vi "stimulate3.vi"(4 "Injection point":T3, 6 "Stimulus":sgl[](array[numeric])=[0.0, 0.0, 0.0, 0.0, 0.0, 0.0] format="%#_3p", 7 "Input 1":sgl[](array[numeric])=[0.0, 0.0, 0.0] format="%#_3p", 8 "Input 0":sgl[](array[numeric])=[0.0, 0.0, 0.0] format="%#_3p", 10 "Parameters":T1={"Stimulus"={"Type"=enum."Off", "Phase"=0.0, "Amplitude"=[0.0, 0.0, 0.0], "Injection point"=enum."Total pose", "Closed loop"=FALSE, "Offset"=[0.0, 0.0, 0.0], "Tip -> world"=TRUE, "Frequency"=0.0, "Length"=0.0}, "Goal Filter A"={"Speedup max"=0.0, "Speedup thresh"=0.15, "Speedup nonlin"=0.0, "Filters"=[]}, "Mode controls"={"Hold"=FALSE, "Cancellation"=FALSE, "Goal filter"=FALSE, "Trigger"=FALSE}, "Manipulator type"=enum."Current piezo", "Manipulator calibration"={"Tool offsets"=[[-1.094526e+33, -1.7368205, -2.1260294e-25]], "Tip light calibration"=[[3.2813332, 0.23462732, 0.17832138, -8265.082], [-0.20249099, 2.693321, -0.28150028, -33565.66], [-0.1458117, 0.68216485, 0.8833545, 26862.188], [-1.1202011e-18, 5.861468e-19, 1.7601345e-18, 1.0]], "Axial filter"={"filter structure"=enum."IIR 2nd Order", "Reverse Coefficients"=[], "Forward Coefficients"=[]}, "Lateral filter"={"filter structure"=enum."IIR 2nd Order", "Reverse Coefficients"=[], "Forward Coefficients"=[]}, "Handle light calibration"=[[0.0, 0.0, -11360.0]], "Base pivots"=[], "Output pivots"=[], "Length center"=0.0, "Workspace height"=[0.0, 0.0, 36200.0], "Workspace diameter"=[0.0, 0.0, 36200.0], "Linearization"=[], "Stack travel"=400.0, "Saturation pos"=375.0}, "Network"={"Remote Host"="", "Send Status"=FALSE, "Send Port"=50, "Recv Commands"=FALSE, "Recv Port"=0}, "Goal Filter B"={"Speedup max"=0.0, "Speedup thresh"=0.0, "Speedup nonlin"=0.0, "Filters"=[]}, "Cancellation"={"KP"=1.0, "KI"=2.0, "KD"=61557.0, "Max vel"=20.0, "Max acc"=61557.0, "Int error limit"=2.0}, "Transition time"=0.0, "Estimation and Feedforward"={"Use Raw Data (ignore Kalman Filter)"=FALSE, "Turn Kalman Filter Off"=FALSE, "Use IMC (if off, PID is used)"=FALSE, "KP"=0.0, "KI"=0.0, "KD"=0.0, "Feedforward Control"=FALSE, "Velocity Gain"=[], "KF input delay"=0}} {"Transition time" format="%_3f"; "Cancellation"."Max acc" format="%#_3p"; "Goal Filter B"."Filters"."V limit range" format="%_3p"; "Goal Filter B"."Filters"."V limit" format="%_3p"; "Goal Filter B"."Filters"."Upper Q" format="%_3f"; "Goal Filter B"."Filters"."Upper Fc" format="%_3p"; "Goal Filter B"."Filters"."Lower Q" format="%_3f"; "Goal Filter B"."Filters"."Scale factor" format="%_3f"; "Goal Filter B"."Filters"."Lower Fc" format="%_3p"; "Goal Filter B"."Speedup nonlin" format="%_3p"; "Goal Filter B"."Speedup thresh" format="%_3p"; "Goal Filter B"."Speedup max" format="%_3p"; "Manipulator calibration"."Saturation pos" format="%#.1f"; "Manipulator calibration"."Stack travel" format="%#.1f"; "Manipulator calibration"."Output pivots" format="%#_6f"; "Manipulator calibration"."Base pivots" format="%#_6f"; "Manipulator calibration"."Handle light calibration" format="%#.1f"; "Manipulator calibration"."Tip light calibration" format="%#.1f"; "Goal Filter A"."Filters"."V limit range" format="%_3p"; "Goal Filter A"."Filters"."V limit" format="%_3p"; "Goal Filter A"."Filters"."Upper Q" format="%_3f"; "Goal Filter A"."Filters"."Upper Fc" format="%_3p"; "Goal Filter A"."Filters"."Lower Q" format="%_3f"; "Goal Filter A"."Filters"."Scale factor" format="%_3f"; "Goal Filter A"."Filters"."Lower Fc" format="%_3p"; "Goal Filter A"."Speedup nonlin" format="%_3p"; "Goal Filter A"."Speedup thresh" format="%_3p"; "Goal Filter A"."Speedup max" format="%_3p"; "Stimulus"."Length" min=0.0 max=100.0 step=100.0 format="%#_4p"; "Stimulus"."Frequency" min=0.0 step=100.0 format="%#_4g"; "Stimulus"."Offset" format="%#_3p"; "Stimulus"."Amplitude" format="%#_3p"; "Stimulus"."Phase" min=-180.0 max=360.0 step=100.0 format="%#.2f"}) -> (0 "Output 1":sgl[](array[numeric]) format="%#_3p", 1 "Output 0":sgl[](array[numeric]) format="%#_3p")   [LabVIEW 2011]
uses:
  injection_point.ctl
  stimulus.ctl
  mode_conrols.ctl
  Micron params.ctl
  asap/labview/testing/probe_calibration.ctl
  host/network_params.ctl
  manipulator_cal.ctl
  cancellation/sq_control_params.ctl
  filtering/goal_loop_parms.ctl
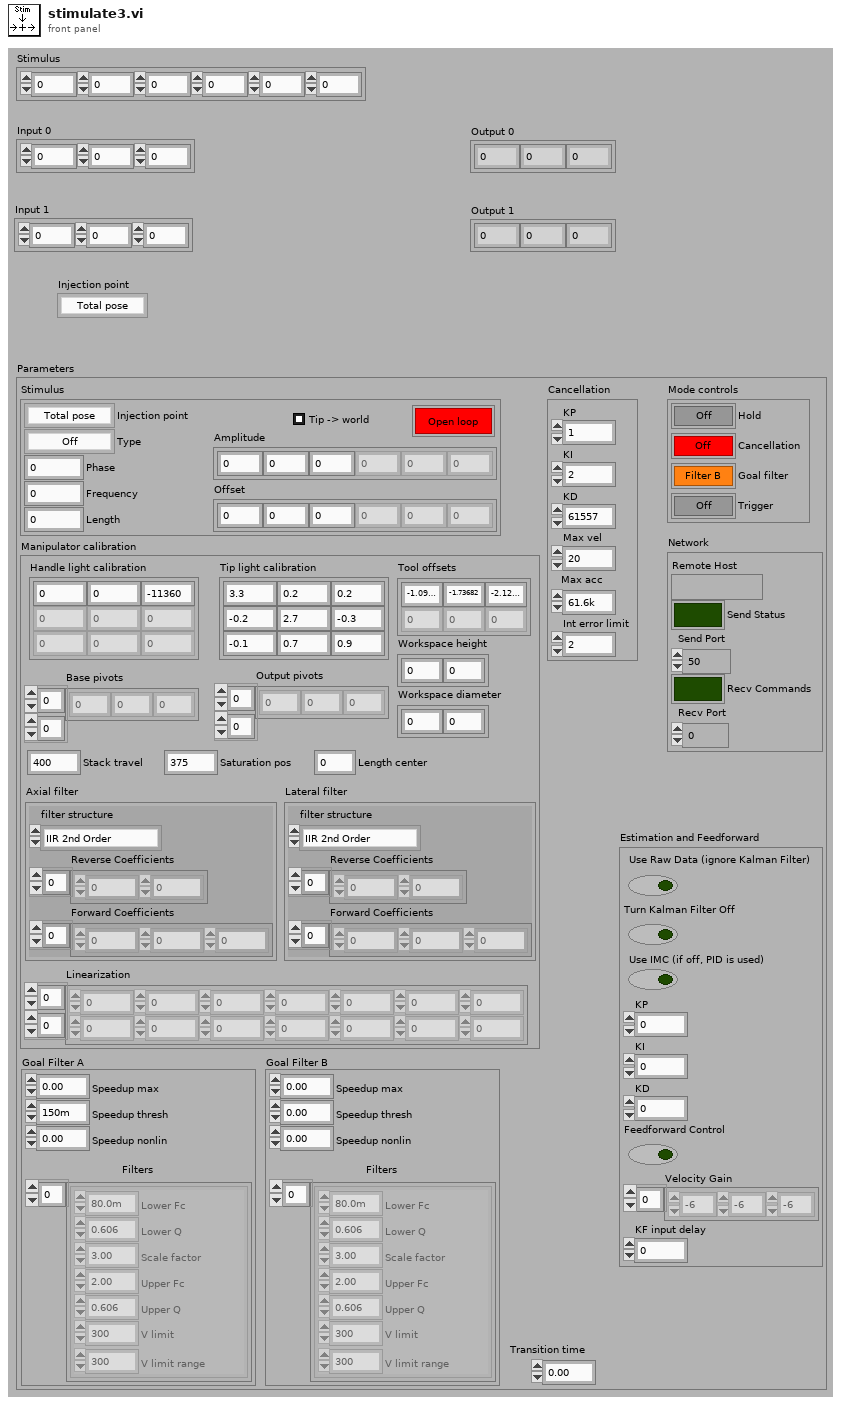
[diagram p1: front panel]
types:
  T1 = typedef "Micron params.ctl" = cluster{"Stimulus":T2, "Goal Filter A":T4, "Mode controls":T5, "Manipulator type":enum16{"Current piezo", "Voltage piezo"}, "Manipulator calibration":T6, "Network":T8, "Goal Filter B":T4, "Cancellation":T9, "Transition time":sgl, "Estimation and Feedforward":cluster{"Use Raw Data (ignore Kalman Filter)":bool, "Turn Kalman Filter Off":bool, "Use IMC (if off, PID is used)":bool, "KP":sgl, "KI":sgl, "KD":sgl, "Feedforward Control":bool, "Velocity Gain":dbl[], "KF input delay":i32}}
  T2 = typedef "stimulus.ctl" = cluster{"Type":enum16{"Off", "Step", "Sine", "Triangle", "Arbitrary"}, "Phase":dbl, "Amplitude":sgl[], "Injection point":T3, "Closed loop":bool, "Offset":sgl[], "Tip -> world":bool, "Frequency":dbl, "Length":dbl}
  T3 = typedef "injection_point.ctl" = enum16{"Total pose", "V limiter", "Goal ", "Link position", "Link rate", "Link residue", "Link goal", "Link error", "Controller", "Output", "Drive", "DAC"}
  T4 = typedef "goal_loop_parms.ctl" = cluster{"Speedup max":sgl, "Speedup thresh":sgl, "Speedup nonlin":sgl, "Filters":cluster{"Lower Fc":sgl, "Lower Q":sgl, "Scale factor":sgl, "Upper Fc":sgl, "Upper Q":sgl, "V limit":sgl, "V limit range":sgl}[]}
  T5 = typedef "mode_conrols.ctl" = cluster{"Hold":bool, "Cancellation":bool, "Goal filter":bool, "Trigger":bool}
  T6 = typedef "manipulator_cal.ctl" = cluster{"Tool offsets":sgl[][], "Tip light calibration":T7, "Axial filter":cluster{"filter structure":enum32{"IIR 2nd Order", "IIR 4th Order"}, "Reverse Coefficients":dbl[], "Forward Coefficients":dbl[]}, "Lateral filter":cluster{"filter structure":enum32{"IIR 2nd Order", "IIR 4th Order"}, "Reverse Coefficients":dbl[], "Forward Coefficients":dbl[]}, "Handle light calibration":T7, "Base pivots":sgl[][], "Output pivots":sgl[][], "Length center":sgl, "Workspace height":sgl[], "Workspace diameter":sgl[], "Linearization":sgl[][], "Stack travel":sgl, "Saturation pos":sgl}
  T7 = typedef "probe_calibration.ctl" = sgl[][]
  T8 = typedef "network_params.ctl" = cluster{"Remote Host":string, "Send Status":bool, "Send Port":u16, "Recv Commands":bool, "Recv Port":u16}
  T9 = typedef "sq_control_params.ctl" = cluster{"KP":sgl, "KI":sgl, "KD":sgl, "Max vel":sgl, "Max acc":sgl, "Int error limit":dbl}
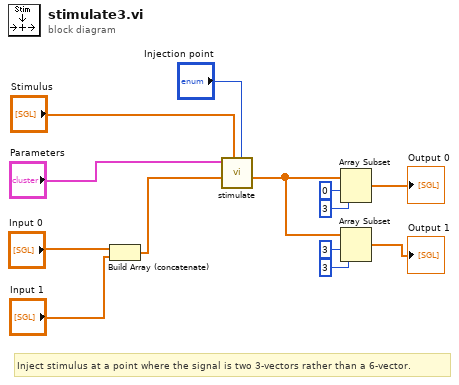
[diagram p0: block diagram]
diagram:
  # "Inject stimulus at a point where the signal is two 3-vectors rather than a 6-vector."
  n1 = Build Array (concatenate)("Input 0", "Input 1") -> (w8:sgl[])
  n2 = call "stimulate.vi"("Injection point"="Injection point", "Stimulus"="Stimulus", "Input"=w8, "Parameters"="Parameters") -> ("Output"=w3:sgl[])  [unwired: 1 in, 5 out]
  n3 = Array Subset(array=w3, index=0, length=3) -> (→"Output 0":sgl[])
  n4 = Array Subset(array=w3, index=3, length=3) -> (→"Output 1":sgl[])
